vi "ActionVIOnCompile.vi"(8 "error in (no error)":errorcluster, 11 "Device Item Ref in":T1 format="%.0x") -> (0 "error out":errorcluster)   [LabVIEW 2013, in "FPGA Addon System Explorer.lvlib"]
uses:
  FPGA Addon System Explorer.lvlib
  <vilib>/NI Veristand/Custom Device API/Custom Device Item Ref.ctl
  <vilib>/NI Veristand/Custom Device API/Data Access Type.ctl
  Shared/FG Action.ctl
  Shared/Compiled.Settings
  Shared/Compiled.RegisterSettings.ctl
  Shared/Scalar Type.ctl
  Shared/Register Information.ctl
  <userlib>/_OpenG.lib/lvdata/lvdata.llb/Type Descriptor Enumeration__ogtk.ctl
  <vilib>/NI Veristand/Custom Device API/Block Data Reference.ctl
  <vilib>/NI Veristand/Custom Device API/Data Reference.ctl
  Shared/Compiled.DMASettings.ctl
  Shared/DMA Settings.ctl
  Shared/Delacing Scheme.ctl
  <vilib>/NI Veristand/Custom Device API/Waveform Data Reference.ctl
  Shared/FPGA Settings.ctl
  Shared/Available Registers FG.vi
  Shared/Constants.vi
  <vilib>/NI Veristand/Custom Device API/Set Item Property (Variant).vi
  <vilib>/NI Veristand/Custom Device API/NI VeriStand - Get Item Property.vi
  <vilib>/NI Veristand/Custom Device API/Get Item Property (Path).vi
  <vilib>/NI Veristand/Custom Device API/Get Item Property (String).vi
  <vilib>/NI Veristand/Custom Device Tools/Custom Device Utility Library/NI VeriStand - Search for Item.vi
  <vilib>/NI Veristand/Custom Device Tools/Custom Device Utility Library/NI VeriStand - Search for Item by GUID.vi
  <vilib>/NI Veristand/Custom Device API/NI VeriStand - Get Item Children.vi
  <vilib>/NI Veristand/Custom Device API/Get Item Property (Variant).vi
  <vilib>/NI VeriStand/Custom Device API/Custom Device API.lvlib
  Shared/FPGA Addon Shared.lvlib
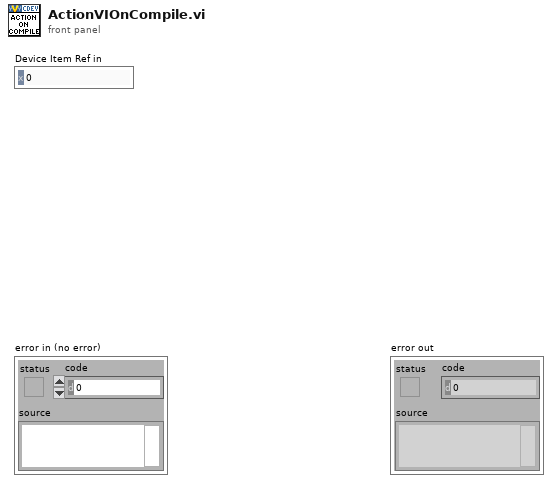
[diagram p1: front panel]
types:
  T1 = typedef "Custom Device API.lvlib/Custom Device Item Ref.ctl" = u64
  T2 = typedef "FPGA Addon Shared.lvlib/Compiled.Settings" = cluster{"Name":string, "IncomingRegisters.Settings":T3[], "IncomingRegisters.Refs":cluster{"Refs":T7[], "Values":dbl[]}, "OutgoingRegisters.Settings":T3[], "OutgoingRegisters.Refs":cluster{"Refs":T7[], "Values":dbl[]}, "Incoming.Size":i32, "Outgoing.Size":i32, "IncomingDMA.Settings":T9[], "OutgoingDMA.Settings":T9[], "FPGA.Settings":T13}
  T3 = typedef "FPGA Addon Shared.lvlib/Compiled.RegisterSettings.ctl" = cluster{"Scalar Type":T4, "Index":i32, "Length":i32, "Register":T5}
  T4 = typedef "FPGA Addon Shared.lvlib/Scalar Type.ctl" = enum16{"Standard", "Bitpacked"}
  T5 = typedef "FPGA Addon Shared.lvlib/Register Information.ctl" = cluster{"Name":string, "Data Type":T6, "Default Value":dbl}
  T6 = typedef "Type Descriptor Enumeration__ogtk.ctl" = enum8{"<Null>", "I8", "I16", "I32", "I64", "U8", "U16", "U32", "U64", "SGL", "DBL", "EXT", "CSG", "CDB", "CXT", "0x0F", "0x10", "0x11", "0x12", "0x13", "0x14", "Enum U8", "Enum U16", "Enum U32", "Enum U64", "SGL PQ", "DBL PQ", "EXT PQ", "CSG PQ", "CDB PQ", "CXT PQ", "0x1F", "0x20", "Boolean", "0x22", "0x23", "0x24", "0x25", "0x26", "0x27", "0x28", "0x29", "0x2A", "0x2B", "0x2C", "0x2D", "0x2E", "0x2F", "String", "0x31", "Path", "Pict", "0x34", "0x35", "0x36", "DAQ", "0x38", "0x39", "0x3A", "0x3B", "0x3C", "0x3D", "0x3E", "0x3F", "Array", "0x41", "0x42", "0x43", "0x44", "0x45", "0x46", "0x47", "0x48", "0x49", "0x4A", "0x4B", "0x4C", "0x4D", "0x4E", "0x4F", "Cluster", "0x51", "0x52", "Variant", "Waveform", "0x55", "0x56", "0x57", "0x58", "0x59", "0x5A", "0x5B", "0x5C", "0x5D", "0x5E", "0x5F", "0x60", "0x61", "0x62", "0x63", "0x64", "0x65", "0x66", "0x67", "0x68", "0x69", "0x6A", "0x6B", "0x6C", "0x6D", "0x6E", "0x6F", "Refnum"}
  T7 = typedef "Custom Device API.lvlib/Block Data Reference.ctl" = cluster{"Data Reference":T8, "Offset":i32, "Length":i32}
  T8 = typedef "Custom Device API.lvlib/Data Reference.ctl" = i32
  T9 = typedef "FPGA Addon Shared.lvlib/Compiled.DMASettings.ctl" = cluster{"Name":string, "DMA.Settings":T10, "DMA.VSRefs":T12[], "WritetoVSEngine.Refs":cluster{"Refs":T8[], "Values":dbl[]}}
  T10 = typedef "FPGA Addon Shared.lvlib/DMA Settings.ctl" = cluster{"Number of Channels":u8, "Delacing Scheme":T11, "Update Rate":u32, "dt":dbl}
  T11 = typedef "FPGA Addon Shared.lvlib/Delacing Scheme.ctl" = enum8{"Interlaced"}
  T12 = typedef "Custom Device API.lvlib/Waveform Data Reference.ctl" = i32
  T13 = typedef "FPGA Addon Shared.lvlib/FPGA Settings.ctl" = cluster{"Bitfile path":path, "RIO Device Address":string}
  T14 = typedef "Custom Device API.lvlib/Data Access Type.ctl" = enum16{"Read", "Write"}
  T15 = typedef "FPGA Addon Shared.lvlib/FG Action.ctl" = enum8{"GET", "SET"}
  T16 = typedef "Custom Device API.lvlib/Custom Device Item Info.ctl" = cluster{"Name":string, "Is Channel":bool, "GUID":string, "Is Waveform":bool}
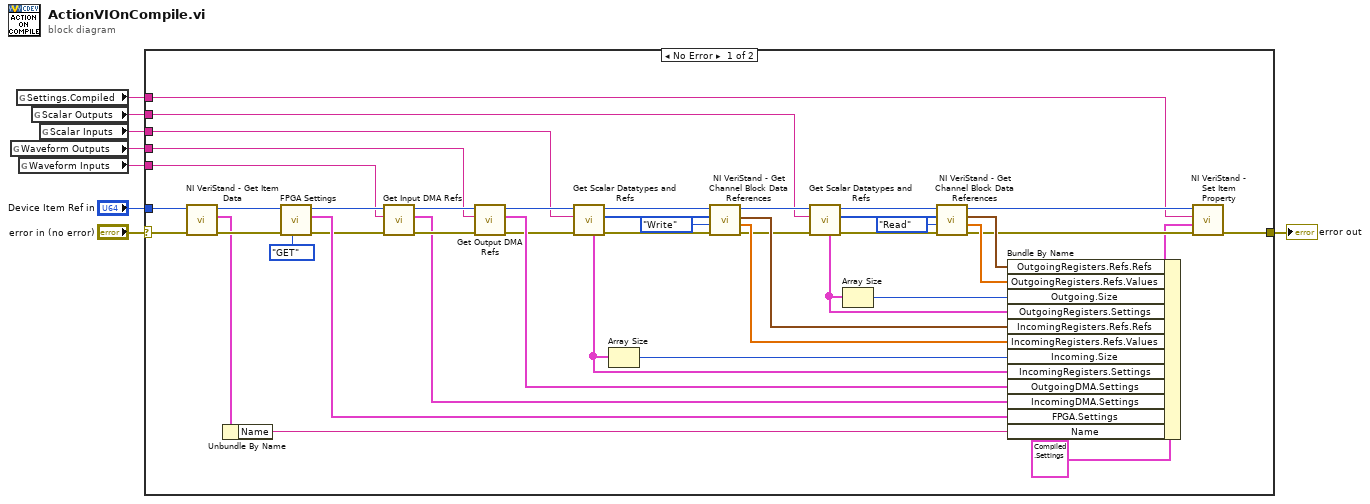
[diagram p0: block diagram]
diagram:
  n1 = global read "Constants.vi" "Waveform Outputs"() -> (w4:string)
  n2 = global read "Constants.vi" "Settings.Compiled"() -> (w1:string)
  n3 = global read "Constants.vi" "Waveform Inputs"() -> (w5:string)
  n4 = global read "Constants.vi" "Scalar Outputs"() -> (w2:string)
  n5 = global read "Constants.vi" "Scalar Inputs"() -> (w3:string)
  n6 = case shown="No Error" "error in (no error)" {
    selector: "error in (no error)" -> [w18 w53]
    tunnel: [w12 w53] -> w7
    tunnel: "Device Item Ref in" -> [w19 _]
    tunnel: w5 -> [w16 _]
    tunnel: w4 -> [w15 _]
    tunnel: w3 -> [w14 _]
    tunnel: w2 -> [w13 _]
    tunnel: w1 -> [w9 _]
    frame No Error {
      n7 = call <vilib>:"NI VeriStand - Get Item Data.vi"("error in (no error)"=w18, "Item Ref in"=w19) -> ("error out"=w50:errorcluster, "Item Info"=w38:T16, "Item Ref out"=w49:T1)  [unwired: 6 in, 1 out]
      n8 = Unbundle By Name(w38) -> ("Name"=w39:string)
      n9 = call "FPGA Settings.vi"("Action"=FG_Action."GET", "error in (no error)"=w50, "Item Ref"=w49) -> ("error out"=w51:errorcluster, "FPGA Settings"=w52:T13, "Item Ref out"=w40:T1)  [unwired: 6 in]
      n10 = call "Get Input DMA Refs.vi"("error in (no error)"=w51, "Item GUID"=w16, "Section Ref in"=w40) -> ("error out"=w42:errorcluster, "DMA Settings"=w41:T9[], "Section Ref out"=w44:T1)  [unwired: 6 in]
      n11 = call "Get Output DMA Refs.vi"("error in (no error)"=w42, "Item GUID"=w15, "Section Ref in"=w44) -> ("error out"=w43:errorcluster, "DMA"=w46:T9[], "Section Ref out"=w45:T1)  [unwired: 6 in]
      n12 = call "Get Scalar Datatypes and Refs.vi"("error in (no error)"=w43, "Item GUID"=w14, "Section Ref in"=w45) -> ("error out"=w23:errorcluster, "VS Ref"=w21:T1[], "Section Ref out"=w22:T1, "Registers Ref"=w47:T3[])  [unwired: 5 in]
      n13 = Array Size(array=w47) -> (size(s)=w36:i32)
      n14 = call <vilib>:"NI VeriStand - Get Channel Block Data References.vi"("error in (no error)"=w23, "Access"=Data_Access_Type."Write", "Channel Refs"=w21, "Device Ref in"=w22) -> ("error out"=w24:errorcluster, "Values Array"=w37:dbl[], "Block Data Refs"=w32:T7[], "Device Ref out"=w25:T1)  [unwired: 4 in]
      n15 = call "Get Scalar Datatypes and Refs.vi"("error in (no error)"=w24, "Item GUID"=w13, "Section Ref in"=w25) -> ("error out"=w27:errorcluster, "VS Ref"=w29:T1[], "Section Ref out"=w28:T1, "Registers Ref"=w48:T3[])  [unwired: 5 in]
      n16 = Array Size(array=w48) -> (size(s)=w35:i32)
      n17 = call <vilib>:"NI VeriStand - Get Channel Block Data References.vi"("error in (no error)"=w27, "Access"=Data_Access_Type."Read", "Channel Refs"=w29, "Device Ref in"=w28) -> ("error out"=w17:errorcluster, "Values Array"=w34:dbl[], "Block Data Refs"=w33:T7[], "Device Ref out"=w10:T1)  [unwired: 4 in]
      n18 = Bundle By Name(cluster=T2 {"Name"="", "IncomingRegisters.Settings"=[], "IncomingRegisters.Refs"={"Refs"=[], "Values"=[]}, "OutgoingRegisters.Settings"=[], "OutgoingRegisters.Refs"={"Refs"=[], "Values"=[]}, "Incoming.Size"=0, "Outgoing.Size"=0, "IncomingDMA.Settings"=[], "OutgoingDMA.Settings"=[], "FPGA.Settings"={"Bitfile path"=path "", "RIO Device Address"=""}}, "OutgoingRegisters.Refs.Refs"=w33, "OutgoingRegisters.Refs.Values"=w34, "Outgoing.Size"=w35, "OutgoingRegisters.Settings"=w48, "IncomingRegisters.Refs.Refs"=w32, "IncomingRegisters.Refs.Values"=w37, "Incoming.Size"=w36, "IncomingRegisters.Settings"=w47, "OutgoingDMA.Settings"=w46, "IncomingDMA.Settings"=w41, "FPGA.Settings"=w52, "Name"=w39) -> (w11:T2)
      n19 = call-poly <vilib>:"NI VeriStand - Set Item Property.vi"("error in (no error)"=w17, "Value"=w11, "Property Name"=w9, "Item Ref in"=w10) -> ("error out"=w12:errorcluster)  [unwired: 5 in, 2 out]
    }
    frame Error {
    }
  }
  "error out" <- w7
